vi "write_params.vi"(8 "error in (no error)":errorcluster, 10 "params":T1={"criterion"="aic", "fit_intercept"=TRUE, "verbose"={"verbose_type"="bool", "verbose_bool"=FALSE, "verbose_int"=0.0}, "normalize"=TRUE, "precompute"={"precompute_type"="auto", "precompute_bool"=FALSE, "precompute_list"=[]}, "max_iter"=500.0, "copy_X"=TRUE, "positive"=FALSE}, 11 "LassoLarsIC in":refnum<class "LassoLarsIC.lvclass">) -> (0 "error out":errorcluster, 3 "LassoLarsIC out":refnum<class "LassoLarsIC.lvclass">)   [LabVIEW 2020, in "LassoLarsIC.lvclass"]
uses:
  LassoLarsIC.lvclass
  Controls/lasso_lars_ic_params.ctl
  LassoLarsIC.lvclass/LassoLarsIC.ctl
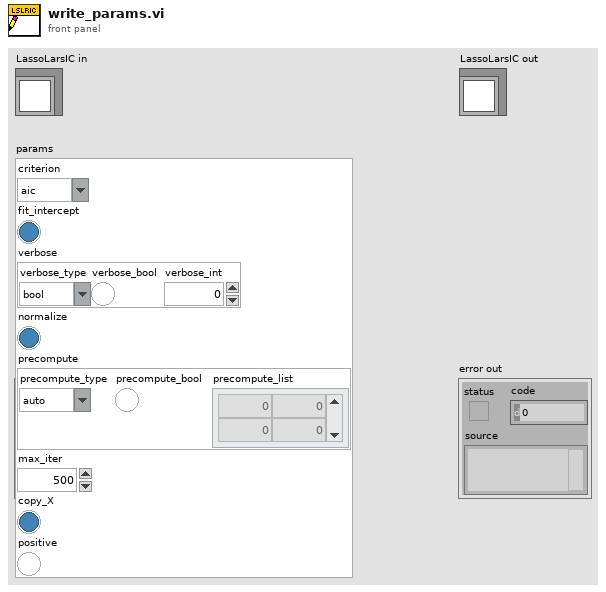
[diagram p1: front panel]
types:
  T1 = typedef "lasso_lars_ic_params.ctl" = cluster{"criterion":string, "fit_intercept":bool, "verbose":cluster{"verbose_type":string, "verbose_bool":bool, "verbose_int":dbl}, "normalize":bool, "precompute":cluster{"precompute_type":string, "precompute_bool":bool, "precompute_list":dbl[][]}, "max_iter":dbl, "copy_X":bool, "positive":bool}
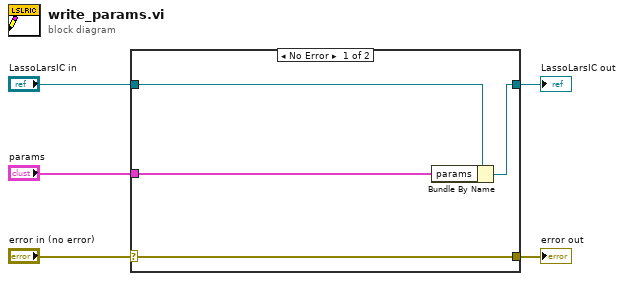
[diagram p0: block diagram]
diagram:
  n1 = case shown="No Error" "error in (no error)" {
    selector: "error in (no error)" -> [w9 w10]
    tunnel: [w9 w10] -> w4
    tunnel: [w7 w11] -> w2
    tunnel: "LassoLarsIC in" -> [w8 w11]
    tunnel: "params" -> [w6 _]
    frame No Error {
      n2 = Bundle By Name(cluster=w8, "params"=w6) -> (w7:refnum<class "LassoLarsIC.lvclass">)
    }
    frame Error {
    }
  }
  "error out" <- w4
  "LassoLarsIC out" <- w2
